vi "VI Tree.vi"   [LabVIEW 2015, in "Rohde&Schwarz CMP LR WPAN Measurement.lvlib"]
doc: "This is the instrument driver for the Rohde&Schwarz CMP LR WPAN Measurement.\nThe VI Tree displays all the user-callable VIs of the instrument driver in an organized table.\n\nFor detailed driver information including modification history, refer to the <B>rscmplrwm.chm</B> file."
uses:
  <instrlib>/Rohde&Schwarz CMP LR WPAN Measurement/Rohde&Schwarz CMP LR WPAN Measurement.lvlib
panel:
  # "rscmplrwm"
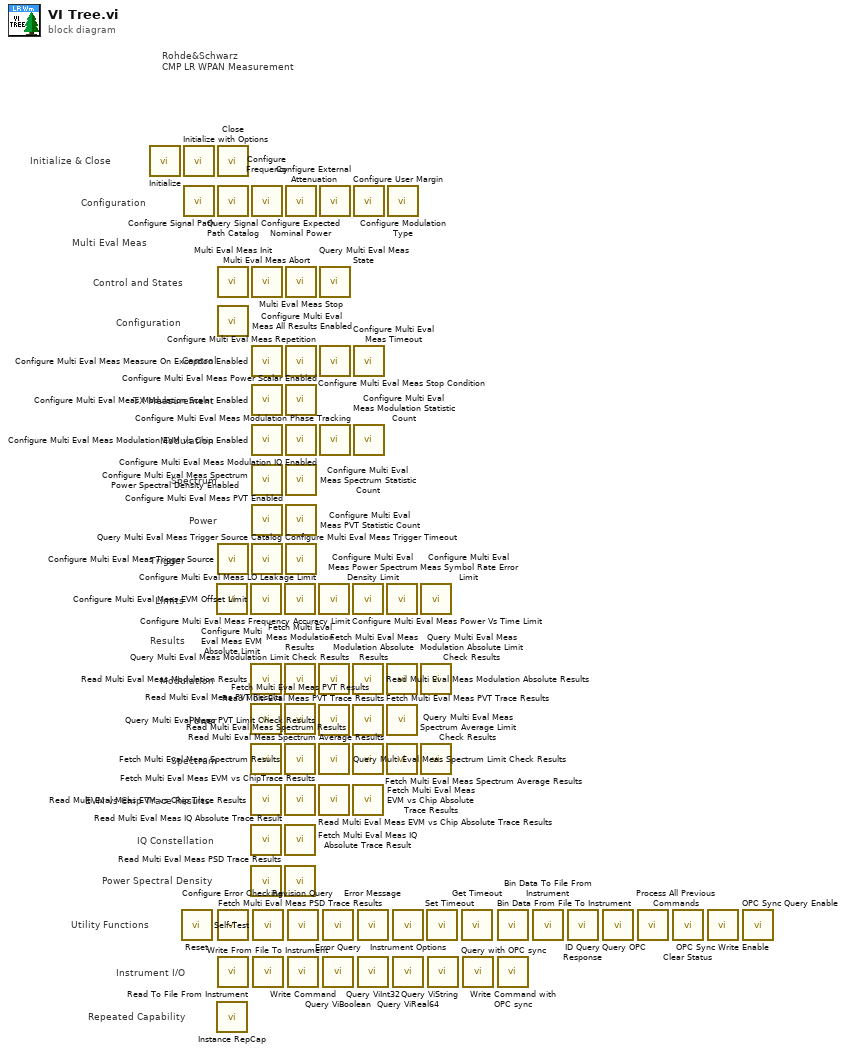
[diagram p0: block diagram]
diagram:
  # "Repeated Capability"
  # "Power Spectral Density"
  # "IQ Constellation"
  # "EVM vs Chip Trace Results"
  # "Spectrum"
  # "Power"
  # "Modulation"
  # "Results"
  # "Limits"
  # "Trigger"
  # "Power"
  # "Spectrum"
  # "Modulation"
  # "TX Measurement"
  # "Control"
  # "Configuration"
  # "Control and States"
  # "Multi Eval Meas"
  # "Configuration"
  # "Rohde&Schwarz\nCMP LR WPAN Measurement"
  # "Instrument I/O"
  # "Utility Functions"
  # "Initialize & Close"
  n1 = call <instrlib>:"Initialize.vi"() -> ()  [unwired: 10 in, 2 out]
  n2 = call <instrlib>:"Reset.vi"() -> ()  [unwired: 10 in, 2 out]
  n3 = call <instrlib>:"Initialize with Options.vi"() -> ()  [unwired: 10 in, 2 out]
  n4 = call <instrlib>:"Configure Signal Path.vi"() -> ()  [unwired: 10 in, 2 out]
  n5 = call <instrlib>:"Configure Multi Eval Meas EVM Absolute Limit.vi"() -> ()  [unwired: 10 in, 2 out]
  n6 = call <instrlib>:"Instance RepCap.vi"() -> ()  [unwired: 2 in, 2 out]
  n7 = call <instrlib>:"Close.vi"() -> ()  [unwired: 11 in, 1 out]
  n8 = call <instrlib>:"Query Signal Path Catalog.vi"() -> ()  [unwired: 9 in, 3 out]
  n9 = call <instrlib>:"Multi Eval Meas Init.vi"() -> ()  [unwired: 10 in, 2 out]
  n10 = call <instrlib>:"Configure Multi Eval Meas All Results Enabled.vi"() -> ()  [unwired: 10 in, 2 out]
  n11 = call <instrlib>:"Configure Multi Eval Meas Trigger Source.vi"() -> ()  [unwired: 10 in, 2 out]
  n12 = call <instrlib>:"Configure Error Checking.vi"() -> ()  [unwired: 10 in, 2 out]
  n13 = call <instrlib>:"Read To File From Instrument.vi"() -> ()  [unwired: 10 in, 2 out]
  n14 = call <instrlib>:"Configure Multi Eval Meas EVM Offset Limit.vi"() -> ()  [unwired: 10 in, 2 out]
  n15 = call <instrlib>:"Read Multi Eval Meas Modulation Results.vi"() -> ()  [unwired: 11 in, 5 out]
  n16 = call <instrlib>:"Read Multi Eval Meas PVT Results.vi"() -> ()  [unwired: 11 in, 5 out]
  n17 = call <instrlib>:"Read Multi Eval Meas Spectrum Results.vi"() -> ()  [unwired: 11 in, 5 out]
  n18 = call <instrlib>:"Read Multi Eval Meas EVM vs Chip Trace Results.vi"() -> ()  [unwired: 8 in, 4 out]
  n19 = call <instrlib>:"Read Multi Eval Meas IQ Absolute Trace Result.vi"() -> ()  [unwired: 11 in, 5 out]
  n20 = call <instrlib>:"Read Multi Eval Meas PSD Trace Results.vi"() -> ()  [unwired: 8 in, 4 out]
  n21 = call <instrlib>:"Configure Frequency.vi"() -> ()  [unwired: 10 in, 2 out]
  n22 = call <instrlib>:"Multi Eval Meas Abort.vi"() -> ()  [unwired: 10 in, 2 out]
  n23 = call <instrlib>:"Configure Multi Eval Meas Measure On Exception Enabled.vi"() -> ()  [unwired: 10 in, 2 out]
  n24 = call <instrlib>:"Configure Multi Eval Meas Modulation Scalar Enabled.vi"() -> ()  [unwired: 10 in, 2 out]
  n25 = call <instrlib>:"Configure Multi Eval Meas Modulation EVM vs Chip Enabled.vi"() -> ()  [unwired: 10 in, 2 out]
  n26 = call <instrlib>:"Configure Multi Eval Meas Spectrum Power Spectral Density Enabled.vi"() -> ()  [unwired: 10 in, 2 out]
  n27 = call <instrlib>:"Configure Multi Eval Meas PVT Enabled.vi"() -> ()  [unwired: 10 in, 2 out]
  n28 = call <instrlib>:"Query Multi Eval Meas Trigger Source Catalog.vi"() -> ()  [unwired: 9 in, 3 out]
  n29 = call <instrlib>:"Self-Test.vi"() -> ()  [unwired: 8 in, 4 out]
  n30 = call <instrlib>:"Write From File To Instrument.vi"() -> ()  [unwired: 10 in, 2 out]
  n31 = call <instrlib>:"Configure Multi Eval Meas LO Leakage Limit.vi"() -> ()  [unwired: 10 in, 2 out]
  n32 = call <instrlib>:"Fetch Multi Eval Meas Modulation Results.vi"() -> ()  [unwired: 11 in, 5 out]
  n33 = call <instrlib>:"Fetch Multi Eval Meas PVT Results.vi"() -> ()  [unwired: 11 in, 5 out]
  n34 = call <instrlib>:"Fetch Multi Eval Meas Spectrum Results.vi"() -> ()  [unwired: 11 in, 5 out]
  n35 = call <instrlib>:"Fetch Multi Eval Meas EVM vs ChipTrace Results.vi"() -> ()  [unwired: 8 in, 4 out]
  n36 = call <instrlib>:"Fetch Multi Eval Meas IQ Absolute Trace Result.vi"() -> ()  [unwired: 11 in, 5 out]
  n37 = call <instrlib>:"Fetch Multi Eval Meas PSD Trace Results.vi"() -> ()  [unwired: 8 in, 4 out]
  n38 = call <instrlib>:"Configure Expected Nominal Power.vi"() -> ()  [unwired: 10 in, 2 out]
  n39 = call <instrlib>:"Multi Eval Meas Stop.vi"() -> ()  [unwired: 10 in, 2 out]
  n40 = call <instrlib>:"Configure Multi Eval Meas Repetition.vi"() -> ()  [unwired: 10 in, 2 out]
  n41 = call <instrlib>:"Configure Multi Eval Meas Power Scalar Enabled.vi"() -> ()  [unwired: 10 in, 2 out]
  n42 = call <instrlib>:"Configure Multi Eval Meas Modulation IQ Enabled.vi"() -> ()  [unwired: 10 in, 2 out]
  n43 = call <instrlib>:"Configure Multi Eval Meas Spectrum Statistic Count.vi"() -> ()  [unwired: 10 in, 2 out]
  n44 = call <instrlib>:"Configure Multi Eval Meas PVT Statistic Count.vi"() -> ()  [unwired: 10 in, 2 out]
  n45 = call <instrlib>:"Configure Multi Eval Meas Trigger Timeout.vi"() -> ()  [unwired: 10 in, 2 out]
  n46 = call <instrlib>:"Revision Query.vi"() -> ()  [unwired: 8 in, 4 out]
  n47 = call <instrlib>:"Write Command.vi"() -> ()  [unwired: 10 in, 2 out]
  n48 = call <instrlib>:"Configure Multi Eval Meas Frequency Accuracy Limit.vi"() -> ()  [unwired: 10 in, 2 out]
  n49 = call <instrlib>:"Query Multi Eval Meas Modulation Limit Check Results.vi"() -> ()  [unwired: 11 in, 5 out]
  n50 = call <instrlib>:"Query Multi Eval Meas PVT Limit Check Results.vi"() -> ()  [unwired: 11 in, 5 out]
  n51 = call <instrlib>:"Query Multi Eval Meas Spectrum Limit Check Results.vi"() -> ()  [unwired: 11 in, 5 out]
  n52 = call <instrlib>:"Read Multi Eval Meas EVM vs Chip Absolute Trace Results.vi"() -> ()  [unwired: 8 in, 4 out]
  n53 = call <instrlib>:"Configure External Attenuation.vi"() -> ()  [unwired: 10 in, 2 out]
  n54 = call <instrlib>:"Query Multi Eval Meas State.vi"() -> ()  [unwired: 7 in, 5 out]
  n55 = call <instrlib>:"Configure Multi Eval Meas Stop Condition.vi"() -> ()  [unwired: 10 in, 2 out]
  n56 = call <instrlib>:"Configure Multi Eval Meas Modulation Phase Tracking.vi"() -> ()  [unwired: 10 in, 2 out]
  n57 = call <instrlib>:"Error Query.vi"() -> ()  [unwired: 8 in, 4 out]
  n58 = call <instrlib>:"Query ViBoolean.vi"() -> ()  [unwired: 9 in, 3 out]
  n59 = call <instrlib>:"Configure Multi Eval Meas Power Vs Time Limit.vi"() -> ()  [unwired: 10 in, 2 out]
  n60 = call <instrlib>:"Read Multi Eval Meas Modulation Absolute Results.vi"() -> ()  [unwired: 11 in, 5 out]
  n61 = call <instrlib>:"Read Multi Eval Meas PVT Trace Results.vi"() -> ()  [unwired: 8 in, 4 out]
  n62 = call <instrlib>:"Read Multi Eval Meas Spectrum Average Results.vi"() -> ()  [unwired: 7 in, 5 out]
  n63 = call <instrlib>:"Fetch Multi Eval Meas EVM vs Chip Absolute Trace Results.vi"() -> ()  [unwired: 8 in, 4 out]
  n64 = call <instrlib>:"Configure User Margin.vi"() -> ()  [unwired: 10 in, 2 out]
  n65 = call <instrlib>:"Configure Multi Eval Meas Timeout.vi"() -> ()  [unwired: 10 in, 2 out]
  n66 = call <instrlib>:"Configure Multi Eval Meas Modulation Statistic Count.vi"() -> ()  [unwired: 10 in, 2 out]
  n67 = call <instrlib>:"Error Message.vi"() -> ()  [unwired: 7 in, 5 out]
  n68 = call <instrlib>:"Query ViInt32.vi"() -> ()  [unwired: 9 in, 3 out]
  n69 = call <instrlib>:"Configure Multi Eval Meas Power Spectrum Density Limit.vi"() -> ()  [unwired: 10 in, 2 out]
  n70 = call <instrlib>:"Fetch Multi Eval Meas Modulation Absolute Results.vi"() -> ()  [unwired: 11 in, 5 out]
  n71 = call <instrlib>:"Fetch Multi Eval Meas PVT Trace Results.vi"() -> ()  [unwired: 8 in, 4 out]
  n72 = call <instrlib>:"Fetch Multi Eval Meas Spectrum Average Results.vi"() -> ()  [unwired: 7 in, 5 out]
  n73 = call <instrlib>:"Configure Modulation Type.vi"() -> ()  [unwired: 10 in, 2 out]
  n74 = call <instrlib>:"Instrument Options.vi"() -> ()  [unwired: 9 in, 3 out]
  n75 = call <instrlib>:"Query ViReal64.vi"() -> ()  [unwired: 9 in, 3 out]
  n76 = call <instrlib>:"Configure Multi Eval Meas Symbol Rate Error Limit.vi"() -> ()  [unwired: 10 in, 2 out]
  n77 = call <instrlib>:"Query Multi Eval Meas Modulation Absolute Limit Check Results.vi"() -> ()  [unwired: 11 in, 5 out]
  n78 = call <instrlib>:"Query Multi Eval Meas Spectrum Average Limit Check Results.vi"() -> ()  [unwired: 7 in, 5 out]
  n79 = call <instrlib>:"Set Timeout.vi"() -> ()  [unwired: 10 in, 2 out]
  n80 = call <instrlib>:"Query ViString.vi"() -> ()  [unwired: 9 in, 3 out]
  n81 = call <instrlib>:"Get Timeout.vi"() -> ()  [unwired: 9 in, 3 out]
  n82 = call <instrlib>:"Query with OPC sync.vi"() -> ()  [unwired: 9 in, 3 out]
  n83 = call <instrlib>:"Bin Data From File To Instrument.vi"() -> ()  [unwired: 10 in, 2 out]
  n84 = call <instrlib>:"Write Command with OPC sync.vi"() -> ()  [unwired: 10 in, 2 out]
  n85 = call <instrlib>:"Bin Data To File From Instrument.vi"() -> ()  [unwired: 10 in, 2 out]
  n86 = call <instrlib>:"ID Query Response.vi"() -> ()  [unwired: 9 in, 3 out]
  n87 = call <instrlib>:"Query OPC.vi"() -> ()  [unwired: 9 in, 3 out]
  n88 = call <instrlib>:"Process All Previous Commands.vi"() -> ()  [unwired: 10 in, 2 out]
  n89 = call <instrlib>:"Clear Status.vi"() -> ()  [unwired: 14 in, 2 out]
  n90 = call <instrlib>:"OPC Sync Write Enable.vi"() -> ()  [unwired: 10 in, 2 out]
  n91 = call <instrlib>:"OPC Sync Query Enable.vi"() -> ()  [unwired: 10 in, 2 out]
